vi "Lab11_LabView.vi"() -> ()   [LabVIEW 2022 SP3]
uses:
  <vilib>/Instr/_visa.llb/VISA Configure Serial Port (Instr).vi
panel:
  in  "stop":bool
  in  "Switch 2":bool
  in  "Switch 1":bool
  in  "VISA resource name":refnum<visa-resource-name>
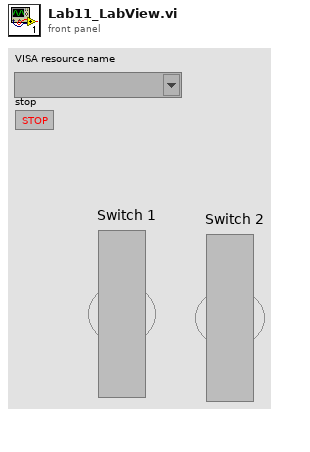
[diagram p1: front panel]
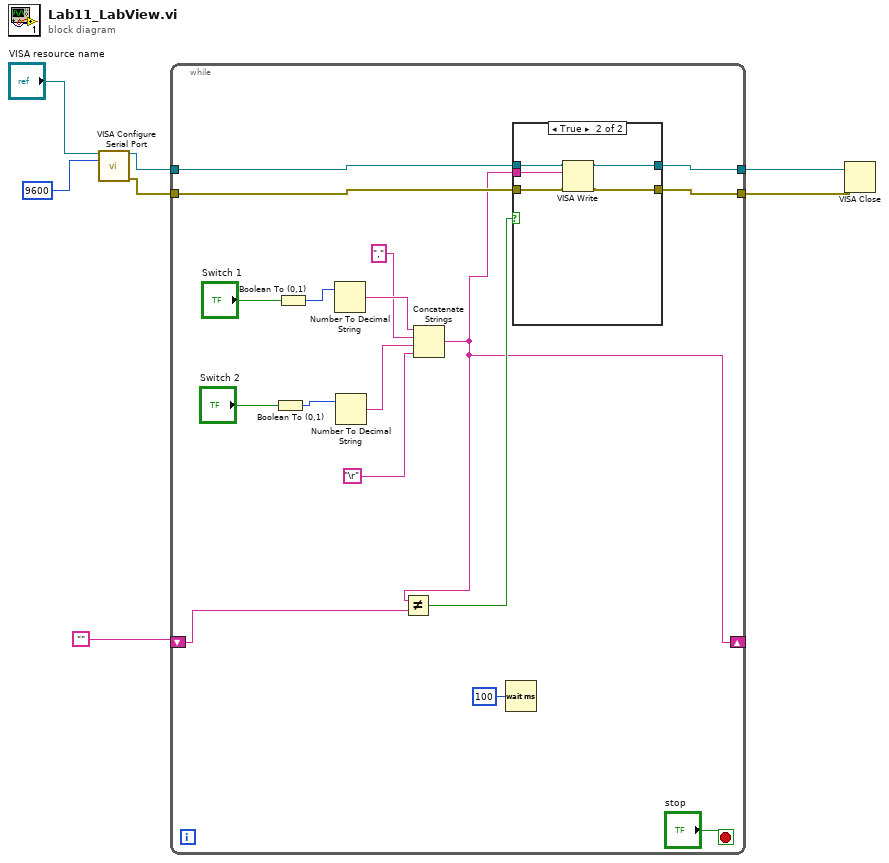
[diagram p0: block diagram]
diagram:
  n1 = call-poly "VISA Configure Serial Port"("VISA resource name"="VISA resource name", "baud rate (9600)"=u32 9600) -> ("VISA resource name out"=w7:refnum<visa-resource-name>, "error out"=w6:errorcluster)  [unwired: 12 in]
  n2 = while {
    tunnel: w7 -> [w16]
    tunnel: w6 -> [w14]
    tunnel: [w13] -> w3
    tunnel: [w15] -> w2
    shift-right: [w10] -> _
    shift-left: "" -> [w12]
    stop <- "stop" stop-if-true
    n3 = Boolean To (0,1)(Boolean="Switch 2") -> (0, 1=w23:i16)
    n4 = Boolean To (0,1)(Boolean="Switch 1") -> (0, 1=w24:i16)
    n5 = Number To Decimal String(number=w24) -> (decimal integer string=w20:string)  [unwired: 1 in]
    n6 = Number To Decimal String(number=w23) -> (decimal integer string=w19:string)  [unwired: 1 in]
    n7 = Concatenate Strings(w20, ",", w19, "\r") -> (w10:string)
    n8 = Not Equal?(x=w10, y=w12) -> (x != y?=w11:bool)
    n9 = Wait (ms)(milliseconds to wait=u32 100) -> ()  [unwired: 1 out]
    n10 = case shown="True" w11 {
      tunnel: w16 -> [w26 w31]
      tunnel: [w26 w30] -> w15
      tunnel: w14 -> [w25 w29]
      tunnel: [w25 w28] -> w13
      tunnel: w10 -> [_ w27]
      frame False {
      }
      frame True {
        n11 = VISA Write(VISA resource name=w31, write buffer=w27, error in (no error)=w29) -> (VISA resource name out=w30:refnum<visa-resource-name>, error out=w28:errorcluster)  [unwired: 1 out]
      }
    }
  }
  n12 = VISA Close(VISA resource name=w2, error in (no error)=w3) -> ()  [unwired: 1 out]
